vi "Verify Data Stream.vi"(6 "Sync Guard Data":fxp<+/-,38,12>[](array[numeric])=[888.2284999489784, 399.7682446986437, -617.0920498371124] format="%.9g", 7 "Elements Remaining In":u32, 8 "error in (no error)":errorcluster, 9 "DataFiltered In":fxp<+/-,38,12>[](array[numeric]), 10 "Data Unfiltered In":fxp<+/-,38,12>[](array[numeric]), 11 "FPGA VI Reference":T1) -> (0 "error out":errorcluster, 1 "DataFiltered Out":fxp<+/-,38,12>[](array[numeric]), 2 "Data Unfiltered Out":fxp<+/-,38,12>[](array[numeric]), 3 "Refnum out":T1, 5 "Elements Remaining":u32)   [LabVIEW 2021]
doc: "Author: Scott Hannahs <sth@magnet.fsu.edu>\nCopyright 2018 Florida State University, All rights reserved."
uses:
  RT Controls/FPGA SCH Digitizer Ref.ctl
  <vilib>/Utility/error.llb/Error Cluster From Error Code.vi
  <vilib>/rvi/errors/niLvFpgaAdjustHostInterfaceError.vi
  <vilib>/rvi/interface/nirviMethod/nirviMethod.xnode
  <vilib>/FPGAPlugInAG/Dynamic/niLvFpga_ReadFifo_Dynamic.vi
  <vilib>/rvi/errors/niLvFpgaMergeErrorWithErrorCode.vi
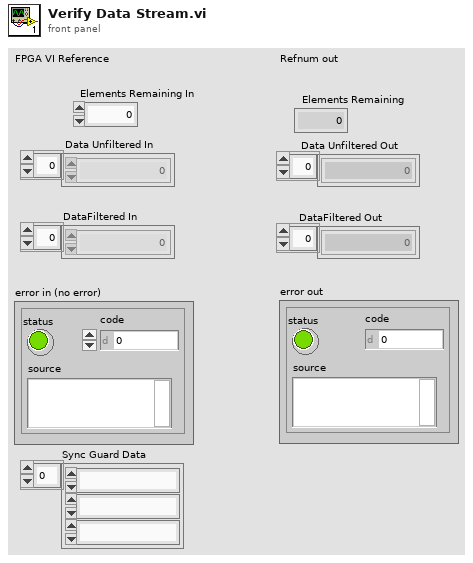
[diagram p1: front panel]
types:
  T1 = typedef "FPGA SCH Digitizer Ref.ctl" = refnum<k20>
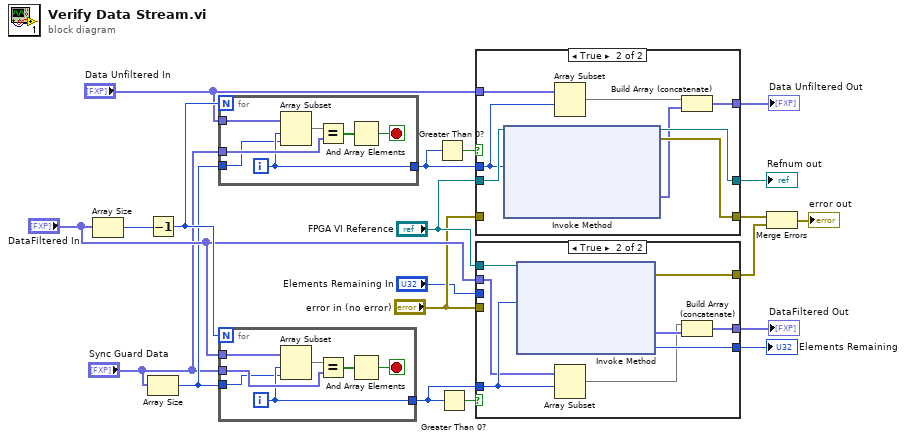
[diagram p0: block diagram]
diagram:
  n1 = Array Size(array="DataFiltered In") -> (size(s)=w20:i32)
  n2 = Decrement(x=w20) -> (x-1=w19:i32)
  n3 = Array Size(array="Sync Guard Data") -> (size(s)=w2:i32)
  n4 = for {
    N: w19 -> [_]
    tunnel: "Data Unfiltered In" -> [w27]
    tunnel: "Sync Guard Data" -> [w25]
    tunnel: [w22] -> w3
    tunnel: w2 -> [w21]
    i -> [w22]
    stop <- w23 stop-if-true
    n5 = Array Subset(array=w27, index=w22, length=w21) -> (w26:fxp<+/-,38,12>[])
    n6 = Equal?(x=w26, y=w25) -> (x = y?=w24:bool[])
    n7 = And Array Elements(Boolean array=w24) -> (logical AND=w23:bool)
  }
  n8 = for {
    N: w19 -> [_]
    tunnel: "DataFiltered In" -> [w34]
    tunnel: "Sync Guard Data" -> [w32]
    tunnel: [w29] -> w4
    tunnel: w2 -> [w28]
    i -> [w29]
    stop <- w30 stop-if-true
    n9 = Array Subset(array=w34, index=w29, length=w28) -> (w33:fxp<+/-,38,12>[])
    n10 = Equal?(x=w33, y=w32) -> (x = y?=w31:bool[])
    n11 = And Array Elements(Boolean array=w31) -> (logical AND=w30:bool)
  }
  n12 = Greater Than 0?(x=w3) -> (x > 0?=w17:bool)
  n13 = Greater Than 0?(x=w4) -> (x > 0?=w18:bool)
  n14 = case shown="True" w17 {
    tunnel: "Data Unfiltered In" -> [w37 w42]
    tunnel: [w37 w39] -> w15
    tunnel: [w36 w45] -> w11
    tunnel: "FPGA VI Reference" -> [w35 w44]
    tunnel: [w35 w43] -> w8
    tunnel: "error in (no error)" -> [w36 _]
    tunnel: w3 -> [_ w40]
    frame False {
    }
    frame True {
      n15 = xnode "Invoke Method"("FPGA VI Reference In"=w44, "Number of Elements"=w40) -> ("FPGA VI Reference Out"=w43:T1, "error out"=w45:errorcluster, "Data"=w38:fxp<+/-,38,12>[])  [unwired: 2 in, 1 out]
      n16 = Array Subset(array=w42, index=w40) -> (w41:fxp<+/-,38,12>[])  [unwired: 1 in]
      n17 = Build Array (concatenate)(w41, w38) -> (w39:fxp<+/-,38,12>[])
    }
  }
  "Refnum out" <- w8
  "Data Unfiltered Out" <- w15
  n18 = case shown="True" w18 {
    tunnel: "DataFiltered In" -> [w47 w50]
    tunnel: [w47 w52] -> w13
    tunnel: [w48 w56] -> w10
    tunnel: "FPGA VI Reference" -> [_ w55]
    tunnel: "error in (no error)" -> [w48 _]
    tunnel: [w46 w54] -> w6
    tunnel: "Elements Remaining In" -> [w46 _]
    tunnel: w4 -> [_ w53]
    frame False {
    }
    frame True {
      n19 = xnode "Invoke Method"("FPGA VI Reference In"=w55, "Number of Elements"=w53) -> ("error out"=w56:errorcluster, "Data"=w51:fxp<+/-,38,12>[], "Elements Remaining"=w54:u32)  [unwired: 2 in, 1 out]
      n20 = Array Subset(array=w50, index=w53) -> (w49:fxp<+/-,38,12>[])  [unwired: 1 in]
      n21 = Build Array (concatenate)(w49, w51) -> (w52:fxp<+/-,38,12>[])
    }
  }
  "DataFiltered Out" <- w13
  "Elements Remaining" <- w6
  n22 = Merge Errors(w11, w10) -> (→"error out":errorcluster)
